vi "Event-Diplom.vi"   [LabVIEW 2018]
uses:
  <vilib>/GPower/UI/Library/GP UI.lvlib
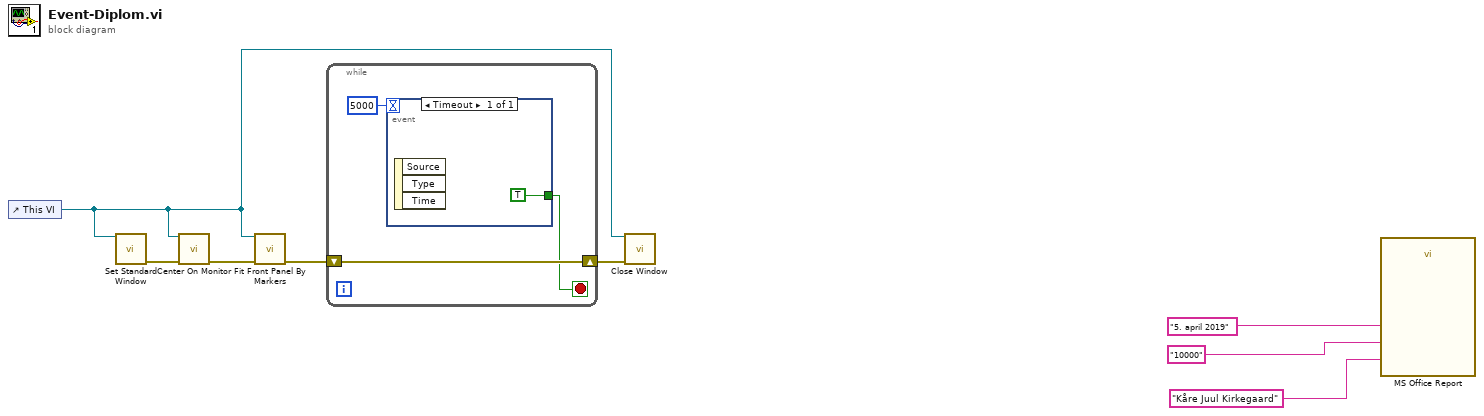
[diagram p0: block diagram]
diagram:
  n1 = control-ref of="This VI"() -> (w4:refnum<vi>)
  n2 = call <vilib>:"Set Standard Window.vi"("VI Refnum"=w4) -> ("Error out"=w6:errorcluster)  [unwired: 14 in]
  n3 = call <vilib>:"Center On Monitor.vi"("VI Refnum"=w4, "Error in"=w6) -> ("Error out"=w5:errorcluster)  [unwired: 13 in]
  n4 = call <vilib>:"Fit Front Panel By Markers.vi"("VI Refnum"=w4, "Error in"=w5) -> ("Error out"=w8:errorcluster)  [unwired: 13 in]
  n5 = while {
    shift-right: [w10] -> w7
    shift-left: w8 -> [w10]
    stop <- w9 stop-if-true
    n6 = event shown="[0] Timeout" {
      selector: _ -> [_]
      dyn-events: _ -> [_]
      timeout: 5000 -> [_]
      tunnel: [TRUE] -> w9
      event Timeout {
        n7 = event-data() -> ()  [unwired: 1 in, 3 out]
      }
    }
  }
  n8 = call <vilib>:"Close Window.vi"("VI Refnum"=w4, "Error in"=w7) -> ()  [unwired: 13 in, 1 out]
  n9 = call "MS Office Report"("Dato"="5. april 2019", "Meter"="10000", "Name"="Kåre Juul Kirkegaard") -> ()  [unwired: 24 in, 1 out]
